vi "NI VeriStand - Set Loop Type.vi"(8 "error in (no error)":errorcluster, 9 "Use Device Clock (Timed Loops only)":bool, 10 "Loop type":T1, 11 "Device Ref in":T2 format="%.0x") -> (0 "error out":errorcluster, 3 "Device Ref out":T2 format="%.0x")   [LabVIEW 2026, in "Custom Devices Storage.lvlib"]
uses:
  Custom Devices Storage.lvlib
  <vilib>/NI VeriStand/Custom Device API/Custom Device Item Ref.ctl
  <vilib>/NI VeriStand/Custom Device API/Custom Device Loop Type.ctl
  C:/Users/Administrator/Desktop/Jatin/All DNC DLLs/NationalInstruments.VeriStand.SystemDefinitionAPI.dll
  Jatin/All DNC DLLs/NationalInstruments.VeriStand.SystemDefinitionAPI.dll
  <vilib>/NI VeriStand/Custom Device API/Custom Device API.lvlib
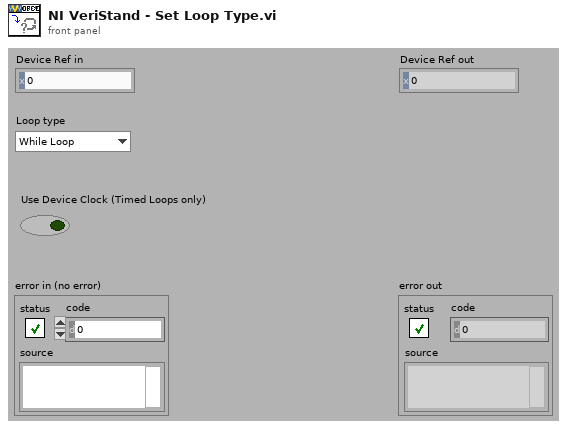
[diagram p1: front panel]
types:
  T1 = typedef "Custom Device API.lvlib/Custom Device Loop Type.ctl" = enum32{"While Loop", "Timed Loop"}
  T2 = typedef "Custom Device API.lvlib/Custom Device Item Ref.ctl" = u64
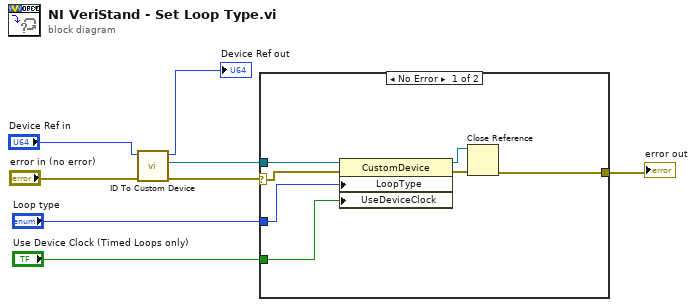
[diagram p0: block diagram]
diagram:
  n1 = call "ID To Custom Device.vi"("error in (no error)"="error in (no error)", "ID in"="Device Ref in") -> ("error out"=w5:errorcluster, "NationalInstruments.VeriStand.SystemDefinitionAPI.CustomDevice"=w4:refnum<k39>, "ID out"=→"Device Ref out":u64)  [unwired: 7 in]
  n2 = case shown="No Error" w5 {
    selector: w5 -> [w14 w16]
    tunnel: w4 -> [w15 _]
    tunnel: "Loop type" -> [w11 _]
    tunnel: "Use Device Clock (Timed Loops only)" -> [w10 _]
    tunnel: [w9 w16] -> w1
    frame No Error {
      n3 = property class="CustomDevice"(reference=w15, error in=w14, "LoopType"=w11, "UseDeviceClock"=w10) -> (reference out=w12:refnum<k39>, error out=w13:errorcluster)
      n4 = Close Reference(reference=w12, error in (no error)=w13) -> (error out=w9:errorcluster)
    }
    frame Error {
    }
  }
  "error out" <- w1
